vi "Open File.vi"(8 "error in (no error)":errorcluster, 11 "Spectrum Recorder in":refnum<class "Spectrum Recorder.lvclass">) -> (0 "error out":errorcluster, 3 "Spectrum Recorder out":refnum<class "Spectrum Recorder.lvclass">)   [LabVIEW 2016, in "Spectrum Recorder.lvclass"]
uses:
  Spectrum Recorder.lvclass
  NHMFL_Core/Libraries/File/Controls/File formats.ctl
  Spectrum Recorder.lvclass/Spectrum Recorder.ctl
  Read Spectrum Recorder Configuration.vi
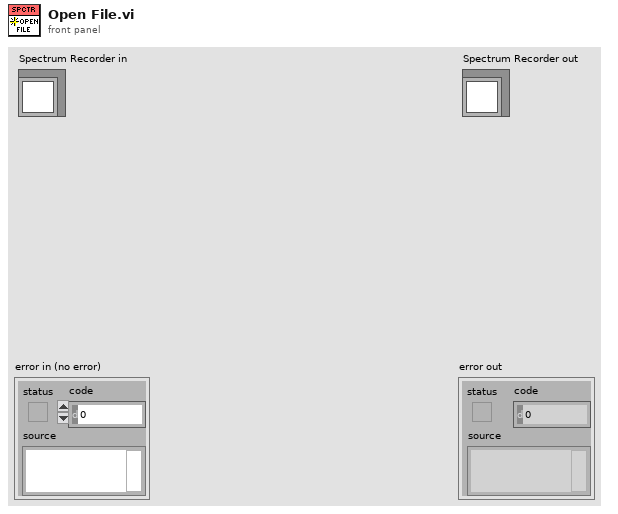
[diagram p1: front panel]
types:
  T1 = enum16{"open", "open or create", "create or replace", "create", "open (read-only)"}
  T2 = typedef "File formats.ctl" = enum16{"TDMS", "ASCII", "BINARY"}
  T3 = typedef "Spectrum Recorder Configuration.ctl" = cluster{"Start":dbl, "End":dbl, "Duration":dbl, "Filter time constant":dbl, "Repeat (-1: forever)":i32, "Update rate":dbl, "Data storage folder":path}
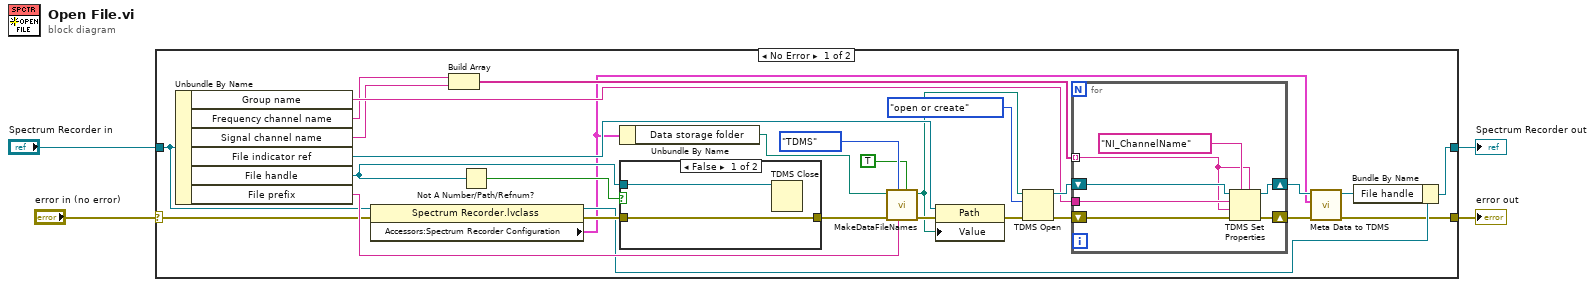
[diagram p0: block diagram]
diagram:
  n1 = case shown="No Error" "error in (no error)" {
    selector: "error in (no error)" -> [w15 w44]
    tunnel: [w5 w44] -> w3
    tunnel: [w25 w43] -> w1
    tunnel: "Spectrum Recorder in" -> [w13 w43]
    frame No Error {
      n2 = Unbundle By Name(w13) -> ("Group name"=w19:string, "Frequency channel name"=w18:string, "Signal channel name"=w10:string, "File indicator ref"=w23:refnum<vi>, "File handle"=w31:refnum<k34>, "File prefix"=w21:string)
      n3 = property class="Spectrum Recorder.lvclass"(reference=w13, error in=w15) -> (reference out=w12:refnum<class "Spectrum Recorder.lvclass">, error out=w14:errorcluster, "Accessors:Spectrum Recorder Configuration"=w7:T3)
      n4 = Build Array(w18, w10) -> (w11:string[])
      n5 = Not A Number/Path/Refnum?(number/path/refnum=w31) -> (NaN/Path/Refnum?=w32:bool)
      n6 = Unbundle By Name(w7) -> ("Data storage folder"=w16:path)
      n7 = case shown="False" w32 {
        tunnel: w31 -> [w41 _]
        tunnel: w14 -> [w40 w42]
        tunnel: [w40 w42] -> w30
        frame False {
          n8 = TDMS Close(11:w41) -> ()  [unwired: 1 in, 2 out]
        }
        frame True {
        }
      }
      n9 = call "MakeDataFileNames.vi"("Include time"=TRUE, "File Prefix"=w21, "File format"=File_formats."TDMS", "Error In"=w30, "Root Data Folder"=w16) -> ("Error Out"=w28:errorcluster, "Data File  Path"=w22:path)  [unwired: 3 in, 2 out]
      n10 = property class="Path"(reference=w23, error in=w28, "Value"=w22) -> (error out=w24:errorcluster)  [unwired: 1 out]
      n11 = TDMS Open(8:w24, 10:T1."open or create" ("operation (0:open)"), 11:w22) -> (0:w17:errorcluster, 3:w20:refnum<k34>)  [unwired: 4 in]
      n12 = for {
        tunnel: w19 -> [w37]
        tunnel: w11 -> [w33] mode=indexing
        shift-right: [w38] -> w9
        shift-left: w20 -> [w39]
        shift-right: [w35] -> w6
        shift-left: w17 -> [w36]
        n13 = TDMS Set Properties(5:w33, 7:"NI_ChannelName", 8:w36, 9:w33, 10:w37, 11:w39) -> (0:w35:errorcluster, 3:w38:refnum<k34>)  [unwired: 2 out]
      }
      n14 = call "Meta Data to TDMS.vi"("Error In"=w6, "Value"=w7, "tdms file"=w9) -> ("Error Out"=w5:errorcluster, "tdms file out"=w8:refnum<k34>)  [unwired: 7 in]
      n15 = Bundle By Name(cluster=w12, "File handle"=w8) -> (w25:refnum<class "Spectrum Recorder.lvclass">)
    }
    frame Error {
    }
  }
  "error out" <- w3
  "Spectrum Recorder out" <- w1
